vi "Begin.vi"(8 "error in":errorcluster) -> (0 "error out":errorcluster)   [LabVIEW 2018]
doc: "Called before other user functions, this VI is expected to open initial I/O refnums, load in file data, and do all program initialization. Notice that the <B>error out</B> terminal is simply used for data flow. Wiring it to other structures or subVIs ensures that this VI runs first."
uses:
  <vilib>/Rock Robotics/WPI/DriverStation/WPI_DriverStationRobotMode2.ctl
  <vilib>/Rock Robotics/WPI/Joystick/WPI_JoystickDeviceEnum.ctl
  <vilib>/Rock Robotics/WPI/ThirdParty/Phoenix-LabVIEW/Motor Controller/Controls/CTRE_Phoenix_MotorControl_NeutralMode.ctl
  <vilib>/Rock Robotics/SystemInterfaces/spilib/spi_bus.ctl
  <vilib>/Rock Robotics/WPI/Solenoid/WPI_SolenoidChannel.ctl
  <vilib>/Rock Robotics/WPI/ThirdParty/Phoenix-LabVIEW/Motor Controller/Controls/CTRE_Phoenix_MotorControl_FeedbackDevice.ctl
  Robot Global Data.vi
  <vilib>/Rock Robotics/Network Tables/NT Write String Array.vi
  <vilib>/Rock Robotics/WPI/Gyro/WPI_GyroXRS450_SPI_Open.vi
  <vilib>/Rock Robotics/WPI/Solenoid/WPI_SolenoidOpenSingle.vi
  <vilib>/Rock Robotics/SystemInterfaces/DIO/FPGA_DIOPWMChannel.ctl
  <vilib>/Rock Robotics/WPI/SafetyOutput/WPI_SafetyOutputConfigMenu.ctl
  <vilib>/Rock Robotics/WPI/RobotDrive/WPI_RobotDriveOpen2MotorWithTalon.vi
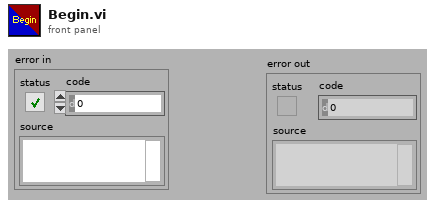
[diagram p1: front panel]
types:
  T1 = typedef "WPI_JoystickDeviceEnum.ctl" = enum16{"USB 0", "USB 1", "USB 2", "USB 3", "USB 4", "USB 5"}
  T2 = typedef "CTRE_Phoenix_MotorControl_FeedbackDevice.ctl" = i8
  T3 = typedef "CTRE_Phoenix_MotorControl_NeutralMode.ctl" = enum8{"EEPROMSetting", "Override to Coast", "Override to Brake"}
  T4 = typedef "WPI_SolenoidChannel.ctl" = enum8{"Solenoid 0", "Solenoid 1", "Solenoid 2", "Solenoid 3", "Solenoid 4", "Solenoid 5", "Solenoid 6", "Solenoid 7", "Invalid"}
  T5 = typedef "spi_bus.ctl" = enum16{"SPI On-Board, CS0", "SPI On-Board, CS1", "SPI On-Board, CS2", "SPI On-Board, CS3", "SPI MXP", "Invalid"}
  T6 = typedef "WPI_DriverStationRobotMode2.ctl" = enum16{"Autonomous Disabled", "Autonomous Enabled", "Teleop Disabled", "Teleop Enabled", "Disconnected", "Finish", "Test Disabled", "Test Enabled", "Emergency Stopped"}
  T7 = typedef "WPI_SafetyOutputConfigMenu.ctl" = enum16{"Enable", "Disable"}
  T8 = typedef "FPGA_DIOPWMChannel.ctl" = enum8{"PWM 0", "PWM 1", "PWM 2", "PWM 3", "PWM 4", "PWM 5", "PWM 6", "PWM 7", "PWM 8", "PWM 9", "PWM MXP 0", "PWM MXP 1", "PWM MXP 2", "PWM MXP 3", "PWM MXP 4", "PWM MXP 5", "PWM MXP 6", "PWM MXP 7", "PWM MXP 8", "PWM MXP 9", "Invalid"}
  T9 = typedef "WPI_RobotDriveDevRef.ctl" = cluster{"DevStatus":errorcluster, "Motors[]":T10[], "Square Inputs":bool, "Max Output":dbl}
  T10 = typedef "WPI_MotorControlDeviceRef.ctl" = cluster{"DeviceStatus":errorcluster, "Type":T11, "PWM":cluster{"PWM Channel":T8, "DeadBand":T12}, "CAN":cluster{"Device Number":u8, "SetOutput VI Ref":variant, "GetOutput VI Ref":variant, "Enable VI Ref":variant, "Disable VI Ref":variant, "Data":variant}, "Invert":bool, "DIO PWM":cluster{"PWM \"Enable\" Channel":T8, "DIOChannel":T13, "PWM Rate":dbl}}
  T11 = typedef "WPI_MotorControlType.ctl" = enum16{"PWM", "CAN", "DIO PWM"}
  T12 = typedef "WPI_PWMDeadband.ctl" = cluster{"Name":string, "maxPositivePwm":i32, "minPositivePwm":i32, "centerPwm":i32, "maxNegativePwm":i32, "minNegativePwm":i32, "angularRange":u16}
  T13 = typedef "FPGA_DIOChannel.ctl" = enum8{"DIO 0", "DIO 1", "DIO 2", "DIO 3", "DIO 4", "DIO 5", "DIO 6", "DIO 7", "DIO 8", "DIO 9", "DIO MXP 0", "DIO MXP 1", "DIO MXP 2", "DIO MXP 3", "DIO MXP 4", "DIO MXP 5", "DIO MXP 6", "DIO MXP 7", "DIO MXP 8", "DIO MXP 9", "DIO MXP 10", "DIO MXP 11", "DIO MXP 12", "DIO MXP 13", "DIO MXP 14", "DIO MXP 15", "SPI Port CS1", "SPI Port CS2", "SPI Port CS3", "SPI Port MISO", "SPI Port MOSI", "Invalid"}
  T14 = typedef "WPI_JoystickDevRef.ctl" = cluster{"Device":T1}
  T15 = typedef "WPI_SolenoidDevRef.ctl" = cluster{"DevStatus":errorcluster, "Pneumatics Control Module":u8, "Forward Solenoid Channel":T4, "Reverse Solenoid Channel":T4}
  T16 = typedef "WPI_GyroDevRef.ctl" = cluster{"DevStatus":errorcluster, "Analog Channel":T17, "Gain (VoltsPerDegree/Second)":dbl, "Gyro Type":enum16{"Analog", "XRS450"}, "Handle":i32, "SPI Bus":T5, "Device Found":bool, "Sample Rate":dbl, "Calibrate On Open":bool, "Offset":dbl}
  T17 = typedef "FPGA_AIChannel.ctl" = enum8{"AI 0", "AI 1", "AI 2", "AI 3", "AI MXP 0", "AI MXP 1", "AI MXP 2", "AI MXP 3", "Invalid"}
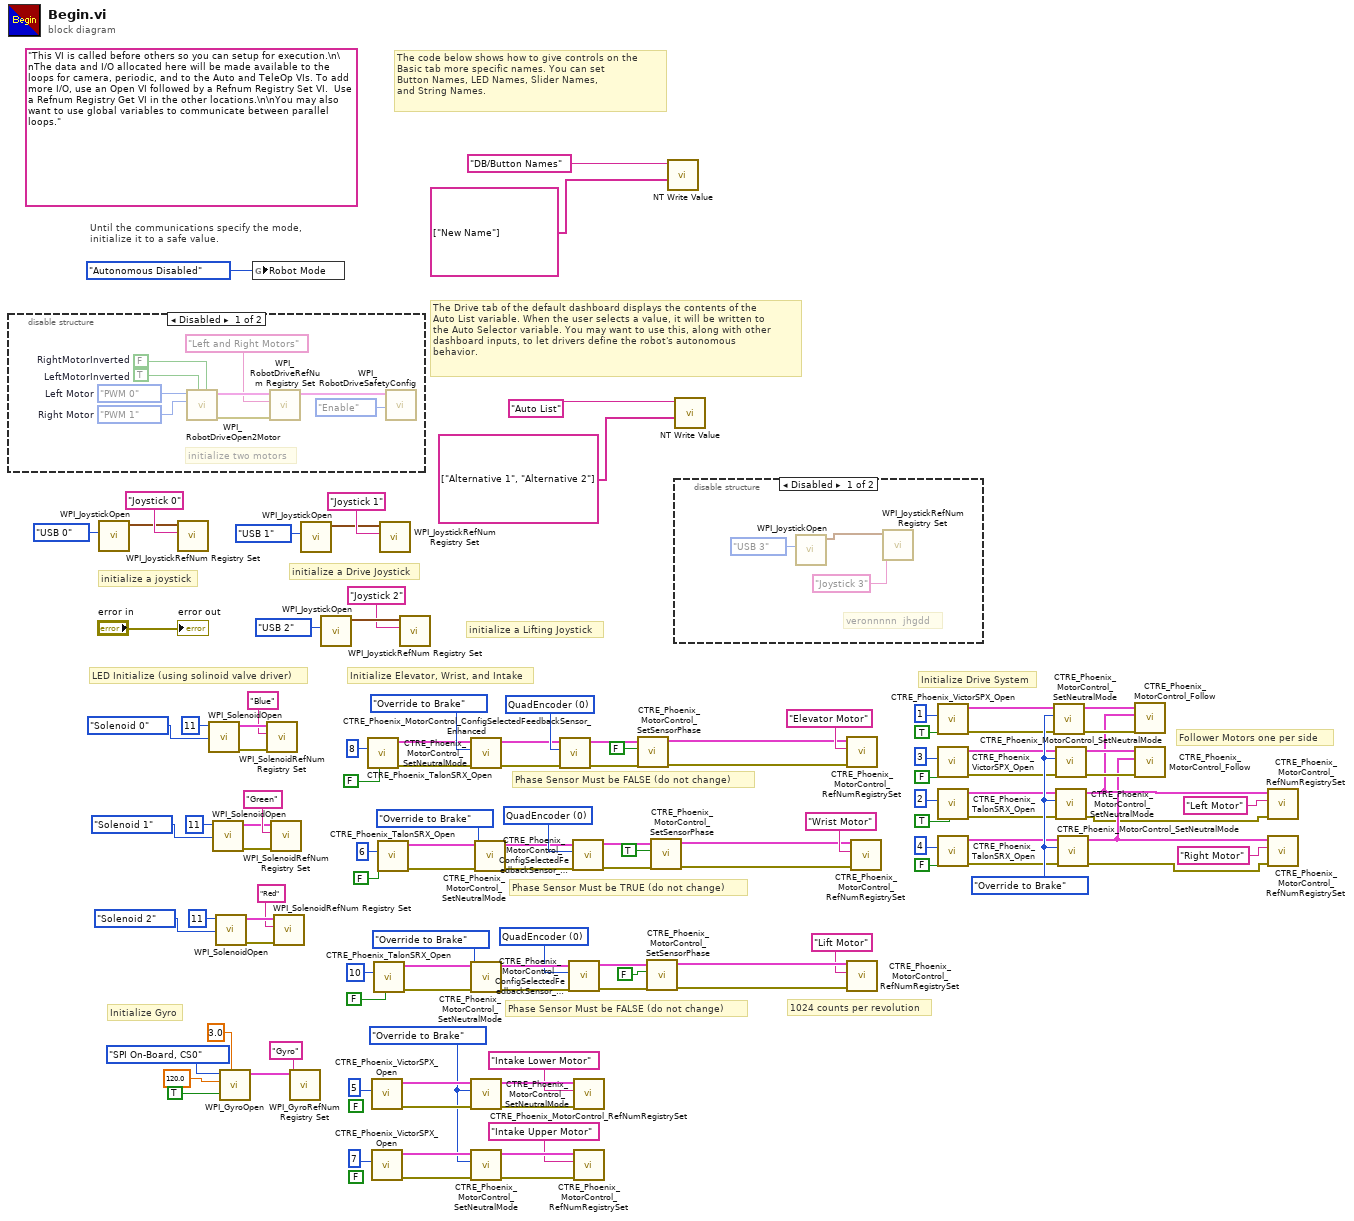
[diagram p0: block diagram]
diagram:
  w12 = T2 0 items=["None"=-1, "QuadEncoder"=0, "Analog"=2, "Tachometer"=4, "Pulse Width Encoded Position"=8, "Sensor Sum (S0 + S1)"=9, "Sensor Difference (D0 - D1)"=10, "Remote Source 0"=11, "Remote Source 1"=12, "Software Emulated"=15] ("Feedback Device")
  w45 = T2 0 items=["None"=-1, "QuadEncoder"=0, "Analog"=2, "Tachometer"=4, "Pulse Width Encoded Position"=8, "Sensor Sum (S0 + S1)"=9, "Sensor Difference (D0 - D1)"=10, "Remote Source 0"=11, "Remote Source 1"=12, "Software Emulated"=15] ("Feedback Device")
  w53 = T2 0 items=["None"=-1, "QuadEncoder"=0, "Analog"=2, "Tachometer"=4, "Pulse Width Encoded Position"=8, "Sensor Sum (S0 + S1)"=9, "Sensor Difference (D0 - D1)"=10, "Remote Source 0"=11, "Remote Source 1"=12, "Software Emulated"=15] ("Feedback Device")
  w78 = CTRE_Phoenix_MotorControl_NeutralMode."Override to Brake" ("Motor Control Neutral Mode")
  (unwired) FALSE ("Invert")
  w89 = CTRE_Phoenix_MotorControl_NeutralMode."Override to Brake" ("Motor Control Neutral Mode")
  (unwired) FALSE ("Invert")
  (unwired) "This VI is called before others so you can setup for execution.\n\nThe data and I/O allocated here will be made available to the loops for camera, periodic, and to the Auto and TeleOp VIs. To add more I/O, use an Open VI followed by a Refnum Registry Set VI.  Use a Refnum Registry Get VI in the other locations.\n\nYou may also want to use global variables to communicate between parallel loops."
  # "1024 counts per revolution"
  # "initialize a Lifting Joystick"
  # "Phase Sensor Must be FALSE (do not change)"
  # "initialize a Drive Joystick"
  # "LED Initialize (using solinoid valve driver)"
  # "Phase Sensor Must be TRUE (do not change)"
  # "Phase Sensor Must be FALSE (do not change)"
  # "Initialize Gyro"
  # "Follower Motors one per side"
  # "Initialize Drive System"
  # "Initialize Elevator, Wrist, and Intake"
  # "The Drive tab of the default dashboard displays the contents of the\nAuto List variable. When the user selects a value, it will be written to\nthe Auto Selector variable. You may want to use this, along with other\ndashboard inputs, to let drivers define the robot's autonomous\nbehavior."
  # "The code below shows how to give controls on the\nBasic tab more specific names. You can set\nButton Names, LED Names, Slider Names,\nand String Names."
  # "initialize a joystick"
  # "Until the communications specify the mode,\ninitialize it to a safe value."
  n1 = disable-structure shown="Disabled" {
    frame Disabled {
      w121 = FPGA_DIOPWMChannel."PWM 1"  # Right Motor
      w122 = FPGA_DIOPWMChannel."PWM 0"  # Left Motor
      w126 = TRUE  # LeftMotorInverted
      w127 = FALSE  # RightMotorInverted
      # "initialize two motors"
      n2 = call-poly <vilib>:"WPI_RobotDriveOpen2Motor.vi"("Right Motor Inverted"=w127, "Left Motor Inverted"=w126, "Right Motor"=w121, "Left Motor"=w122) -> ("error out"=w123:errorcluster, "RobotDriveDevRef"=w125:T9)  [unwired: 1 in, 5 out]
      n3 = call <vilib>:"WPI_RobotDriveRefNum Registry Set.vi"("error in (no error)"=w123, "refnum name"="Left and Right Motors", "RobotDriveDevRef"=w125) -> ("RobotDriveDevRef"=w120:T9)  [unwired: 1 in, 7 out]
      n4 = call <vilib>:"WPI_RobotDriveSafetyConfig.vi"("mode"=WPI_SafetyOutputConfigMenu."Enable", "RobotDriveDevRef"=w120) -> ()  [unwired: 8 in, 2 out]
    }
    frame Enabled {
    }
  }
  n5 = call <vilib>:"WPI_JoystickOpen.vi"("JoystickDevice"=WPI_JoystickDeviceEnum."USB 0") -> ("JoystickDevRef"=w116:T14)  [unwired: 10 in]
  n6 = call <vilib>:"WPI_JoystickRefNum Registry Set.vi"("refnum name"="Joystick 0", "JoystickDevRef"=w116) -> ()  [unwired: 8 in, 2 out]
  n7 = call-poly <vilib>:"WPI_SolenoidOpen.vi"("Solenoid Channel"=WPI_SolenoidChannel."Solenoid 0", "Pneumatics Control Module (0)"=u8 11) -> ("error out"=w35:errorcluster, "SolenoidDevRef"=w34:T15)  [unwired: 8 in]
  n8 = call-poly <vilib>:"WPI_SolenoidOpen.vi"("Solenoid Channel"=WPI_SolenoidChannel."Solenoid 1", "Pneumatics Control Module (0)"=u8 11) -> ("error out"=w30:errorcluster, "SolenoidDevRef"=w31:T15)  [unwired: 8 in]
  n9 = call-poly <vilib>:"WPI_SolenoidOpen.vi"("Solenoid Channel"=WPI_SolenoidChannel."Solenoid 2", "Pneumatics Control Module (0)"=u8 11) -> ("error out"=w25:errorcluster, "SolenoidDevRef"=w24:T15)  [unwired: 8 in]
  n10 = call-poly <vilib>:"WPI_GyroOpen.vi"("Calibration Time (s)"=3.0, "Calibrate On Open"=TRUE, "Sample Rate (Hz)"=120.0, "SPI Bus"=spi_bus."SPI On-Board, CS0") -> ("GyroDevRef"=w55:T16)  [unwired: 5 in, 2 out]
  n11 = global write "Robot Global Data.vi" "Robot Mode"(WPI_DriverStationRobotMode2."Autonomous Disabled" ("Robot Mode")) -> ()
  n12 = call <vilib>:"WPI_SolenoidRefNum Registry Set.vi"("error in (no error)"=w35, "refnum name"="Blue", "SolenoidDevRef"=w34) -> ()  [unwired: 7 in, 2 out]
  n13 = call <vilib>:"WPI_SolenoidRefNum Registry Set.vi"("error in (no error)"=w30, "refnum name"="Green", "SolenoidDevRef"=w31) -> ()  [unwired: 7 in, 2 out]
  n14 = call <vilib>:"WPI_SolenoidRefNum Registry Set.vi"("error in (no error)"=w25, "refnum name"="Red", "SolenoidDevRef"=w24) -> ()  [unwired: 7 in, 2 out]
  n15 = call <vilib>:"WPI_GyroRefNum Registry Set.vi"("refnum name"="Gyro", "GyroDevRef"=w55) -> ()  [unwired: 8 in, 2 out]
  n16 = call <vilib>:"WPI_JoystickOpen.vi"("JoystickDevice"=WPI_JoystickDeviceEnum."USB 1") -> ("JoystickDevRef"=w21:T14)  [unwired: 10 in]
  n17 = call <vilib>:"WPI_JoystickOpen.vi"("JoystickDevice"=WPI_JoystickDeviceEnum."USB 2") -> ("JoystickDevRef"=w5:T14)  [unwired: 10 in]
  n18 = call <vilib>:"CTRE_Phoenix_TalonSRX_Open.vi"("Invert"=FALSE, "Device Number"=u8 8) -> ("error out"=w105:errorcluster, "CAN Talon SRX Ref"=w106:T10)  [unwired: 8 in]
  n19 = call <vilib>:"CTRE_Phoenix_VictorSPX_Open.vi"("Device Number"=u8 5) -> ("error out"=w97:errorcluster, "CAN Talon SRX Ref"=w98:T10)  [unwired: 9 in]
  n20 = call <vilib>:"CTRE_Phoenix_VictorSPX_Open.vi"("Device Number"=u8 7) -> ("error out"=w93:errorcluster, "CAN Talon SRX Ref"=w94:T10)  [unwired: 9 in]
  n21 = call <vilib>:"CTRE_Phoenix_TalonSRX_Open.vi"("Invert"=FALSE, "Device Number"=u8 10) -> ("error out"=w11:errorcluster, "CAN Talon SRX Ref"=w10:T10)  [unwired: 8 in]
  n22 = call <vilib>:"CTRE_Phoenix_TalonSRX_Open.vi"("Invert"=FALSE, "Device Number"=u8 6) -> ("error out"=w100:errorcluster, "CAN Talon SRX Ref"=w101:T10)  [unwired: 8 in]
  n23 = call <vilib>:"WPI_JoystickRefNum Registry Set.vi"("refnum name"="Joystick 1", "JoystickDevRef"=w21) -> ()  [unwired: 8 in, 2 out]
  n24 = call <vilib>:"WPI_JoystickRefNum Registry Set.vi"("refnum name"="Joystick 2", "JoystickDevRef"=w5) -> ()  [unwired: 8 in, 2 out]
  n25 = call <vilib>:"CTRE_Phoenix_MotorControl_SetNeutralMode.vi"("error in (no error)"=w105, "Motor Control Neutral Mode"=CTRE_Phoenix_MotorControl_NeutralMode."Override to Brake", "PhoenixMotorControlDevRef"=w106) -> ("error out"=w48:errorcluster, "PhoenixMotorControlDevRef"=w49:T10)  [unwired: 7 in]
  n26 = call <vilib>:"CTRE_Phoenix_MotorControl_SetNeutralMode.vi"("error in (no error)"=w11, "Motor Control Neutral Mode"=CTRE_Phoenix_MotorControl_NeutralMode."Override to Brake", "PhoenixMotorControlDevRef"=w10) -> ("error out"=w17:errorcluster, "PhoenixMotorControlDevRef"=w16:T10)  [unwired: 7 in]
  n27 = call <vilib>:"CTRE_Phoenix_MotorControl_SetNeutralMode.vi"("error in (no error)"=w97, "Motor Control Neutral Mode"=w89, "PhoenixMotorControlDevRef"=w98) -> ("error out"=w88:errorcluster, "PhoenixMotorControlDevRef"=w99:T10)  [unwired: 7 in]
  n28 = call <vilib>:"CTRE_Phoenix_MotorControl_SetNeutralMode.vi"("error in (no error)"=w93, "Motor Control Neutral Mode"=w89, "PhoenixMotorControlDevRef"=w94) -> ("error out"=w87:errorcluster, "PhoenixMotorControlDevRef"=w95:T10)  [unwired: 7 in]
  n29 = call <vilib>:"CTRE_Phoenix_MotorControl_SetNeutralMode.vi"("error in (no error)"=w100, "Motor Control Neutral Mode"=CTRE_Phoenix_MotorControl_NeutralMode."Override to Brake", "PhoenixMotorControlDevRef"=w101) -> ("error out"=w40:errorcluster, "PhoenixMotorControlDevRef"=w41:T10)  [unwired: 7 in]
  n30 = call <vilib>:"CTRE_Phoenix_MotorControl_ConfigSelectedFeedbackSensor_Enhanced.vi"("error in (no error)"=w48, "Feedback Device"=w53, "PhoenixMotorControlDevRef"=w49) -> ("error out"=w50:errorcluster, "PhoenixMotorControlDevRef"=w51:T10)  [unwired: 7 in]
  n31 = call <vilib>:"CTRE_Phoenix_MotorControl_ConfigSelectedFeedbackSensor_Enhanced.vi"("error in (no error)"=w17, "Feedback Device"=w12, "PhoenixMotorControlDevRef"=w16) -> ("error out"=w15:errorcluster, "PhoenixMotorControlDevRef"=w14:T10)  [unwired: 7 in]
  n32 = call <vilib>:"CTRE_Phoenix_MotorControl_ConfigSelectedFeedbackSensor_Enhanced.vi"("error in (no error)"=w40, "Feedback Device"=w45, "PhoenixMotorControlDevRef"=w41) -> ("error out"=w42:errorcluster, "PhoenixMotorControlDevRef"=w43:T10)  [unwired: 7 in]
  n33 = call <vilib>:"CTRE_Phoenix_MotorControl_RefNumRegistrySet.vi"("error in (no error)"=w88, "refnum name"="Intake Lower Motor", "PhoenixMotorControlDevRef"=w99) -> ()  [unwired: 7 in, 2 out]
  n34 = call <vilib>:"CTRE_Phoenix_MotorControl_RefNumRegistrySet.vi"("error in (no error)"=w87, "refnum name"="Intake Upper Motor", "PhoenixMotorControlDevRef"=w95) -> ()  [unwired: 7 in, 2 out]
  n35 = call <vilib>:"CTRE_Phoenix_MotorControl_SetSensorPhase.vi"("error in (no error)"=w50, "PhaseSensor"=FALSE ("Flip Sensor Elevator"), "PhoenixMotorControlDevRef"=w51) -> ("error out"=w46:errorcluster, "PhoenixMotorControlDevRef"=w47:T10)  [unwired: 7 in]
  n36 = call <vilib>:"CTRE_Phoenix_MotorControl_SetSensorPhase.vi"("error in (no error)"=w15, "PhaseSensor"=FALSE ("Flip Sensor Elevator 2"), "PhoenixMotorControlDevRef"=w14) -> ("error out"=w19:errorcluster, "PhoenixMotorControlDevRef"=w18:T10)  [unwired: 7 in]
  n37 = call <vilib>:"CTRE_Phoenix_MotorControl_SetSensorPhase.vi"("error in (no error)"=w42, "PhaseSensor"=TRUE ("Flip Sensor Elevator 2"), "PhoenixMotorControlDevRef"=w43) -> ("error out"=w38:errorcluster, "PhoenixMotorControlDevRef"=w39:T10)  [unwired: 7 in]
  n38 = call-poly <vilib>:"NT Write Value.vi"("String Array"=string[] ["New Name"], "Name"="DB/Button Names") -> ()  [unwired: 9 in, 1 out]
  n39 = call-poly <vilib>:"NT Write Value.vi"("String Array"=string[] ["Alternative 1", "Alternative 2"], "Name"="Auto List") -> ()  [unwired: 9 in, 1 out]
  n40 = disable-structure shown="Disabled" {
    frame Disabled {
      # "veronnnnn  jhgdd"
      n41 = call <vilib>:"WPI_JoystickOpen.vi"("JoystickDevice"=WPI_JoystickDeviceEnum."USB 3") -> ("JoystickDevRef"=w129:T14)  [unwired: 10 in]
      n42 = call <vilib>:"WPI_JoystickRefNum Registry Set.vi"("refnum name"="Joystick 3", "JoystickDevRef"=w129) -> ()  [unwired: 8 in, 2 out]
    }
    frame Enabled {
    }
  }
  n43 = call <vilib>:"CTRE_Phoenix_MotorControl_RefNumRegistrySet.vi"("error in (no error)"=w46, "refnum name"="Elevator Motor", "PhoenixMotorControlDevRef"=w47) -> ()  [unwired: 7 in, 2 out]
  n44 = call <vilib>:"CTRE_Phoenix_MotorControl_RefNumRegistrySet.vi"("error in (no error)"=w19, "refnum name"="Lift Motor", "PhoenixMotorControlDevRef"=w18) -> ()  [unwired: 7 in, 2 out]
  n45 = call <vilib>:"CTRE_Phoenix_MotorControl_RefNumRegistrySet.vi"("error in (no error)"=w38, "refnum name"="Wrist Motor", "PhoenixMotorControlDevRef"=w39) -> ()  [unwired: 7 in, 2 out]
  n46 = call <vilib>:"CTRE_Phoenix_VictorSPX_Open.vi"("Invert"=TRUE, "Device Number"=u8 1) -> ("error out"=w73:errorcluster, "CAN Talon SRX Ref"=w77:T10)  [unwired: 8 in]
  n47 = call <vilib>:"CTRE_Phoenix_VictorSPX_Open.vi"("Invert"=FALSE, "Device Number"=u8 3) -> ("error out"=w71:errorcluster, "CAN Talon SRX Ref"=w76:T10)  [unwired: 8 in]
  n48 = call <vilib>:"CTRE_Phoenix_TalonSRX_Open.vi"("Invert"=TRUE, "Device Number"=u8 2) -> ("error out"=w63:errorcluster, "CAN Talon SRX Ref"=w65:T10)  [unwired: 8 in]
  n49 = call <vilib>:"CTRE_Phoenix_TalonSRX_Open.vi"("Invert"=FALSE, "Device Number"=u8 4) -> ("error out"=w62:errorcluster, "CAN Talon SRX Ref"=w64:T10)  [unwired: 8 in]
  n50 = call <vilib>:"CTRE_Phoenix_MotorControl_SetNeutralMode.vi"("error in (no error)"=w73, "Motor Control Neutral Mode"=w78, "PhoenixMotorControlDevRef"=w77) -> ("error out"=w72:errorcluster, "PhoenixMotorControlDevRef"=w75:T10)  [unwired: 7 in]
  n51 = call <vilib>:"CTRE_Phoenix_MotorControl_SetNeutralMode.vi"("error in (no error)"=w71, "Motor Control Neutral Mode"=w78, "PhoenixMotorControlDevRef"=w76) -> ("error out"=w70:errorcluster, "PhoenixMotorControlDevRef"=w74:T10)  [unwired: 7 in]
  n52 = call <vilib>:"CTRE_Phoenix_MotorControl_SetNeutralMode.vi"("error in (no error)"=w63, "Motor Control Neutral Mode"=w78, "PhoenixMotorControlDevRef"=w65) -> ("error out"=w61:errorcluster, "PhoenixMotorControlDevRef"=w68:T10)  [unwired: 7 in]
  n53 = call <vilib>:"CTRE_Phoenix_MotorControl_SetNeutralMode.vi"("error in (no error)"=w62, "Motor Control Neutral Mode"=w78, "PhoenixMotorControlDevRef"=w64) -> ("error out"=w60:errorcluster, "PhoenixMotorControlDevRef"=w66:T10)  [unwired: 7 in]
  n54 = call <vilib>:"CTRE_Phoenix_MotorControl_Follow.vi"("error in (no error)"=w72, "Master Controller to Follow"=w68, "PhoenixMotorControlDevRef"=w75) -> ()  [unwired: 7 in, 2 out]
  n55 = call <vilib>:"CTRE_Phoenix_MotorControl_Follow.vi"("error in (no error)"=w70, "Master Controller to Follow"=w66, "PhoenixMotorControlDevRef"=w74) -> ()  [unwired: 7 in, 2 out]
  n56 = call <vilib>:"CTRE_Phoenix_MotorControl_RefNumRegistrySet.vi"("error in (no error)"=w61, "refnum name"="Left Motor", "PhoenixMotorControlDevRef"=w68) -> ()  [unwired: 7 in, 2 out]
  n57 = call <vilib>:"CTRE_Phoenix_MotorControl_RefNumRegistrySet.vi"("error in (no error)"=w60, "refnum name"="Right Motor", "PhoenixMotorControlDevRef"=w66) -> ()  [unwired: 7 in, 2 out]
  "error out" <- "error in"
